vi "Test.vi"() -> ()   [LabVIEW 2013]
uses:
  <resource>/Framework/Providers/lveio/public/EIOAttr.ctl
panel:
  out "Type GUID 2":string
  out "Type GUID":string
  out "Type String 2":string
  out "Array 2":string[](array[string])
  out "properties":T1[](array[typedef])
  out "Array":string[](array[string])
  out "Value":variant
  out "Is Persistent":bool
  out "Tag:Get Names":string[](array[string])
  out "Type String":string
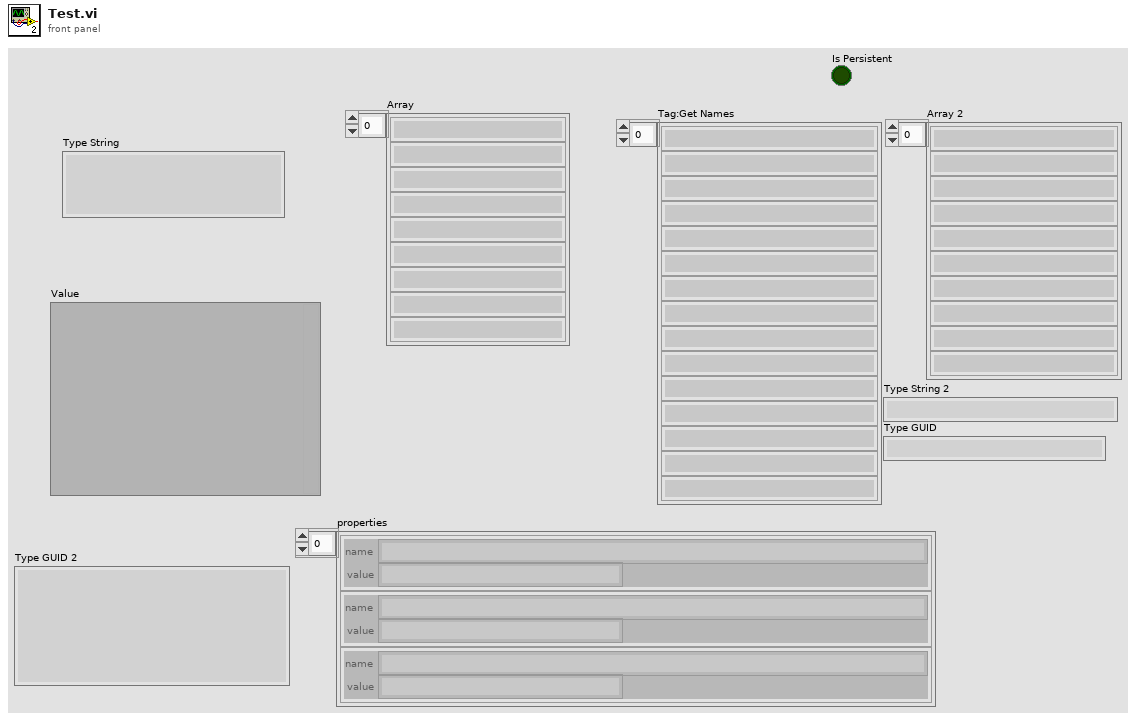
[diagram p1: front panel]
types:
  T1 = typedef "EIOAttr.ctl" = cluster{"name":string, "value":string}
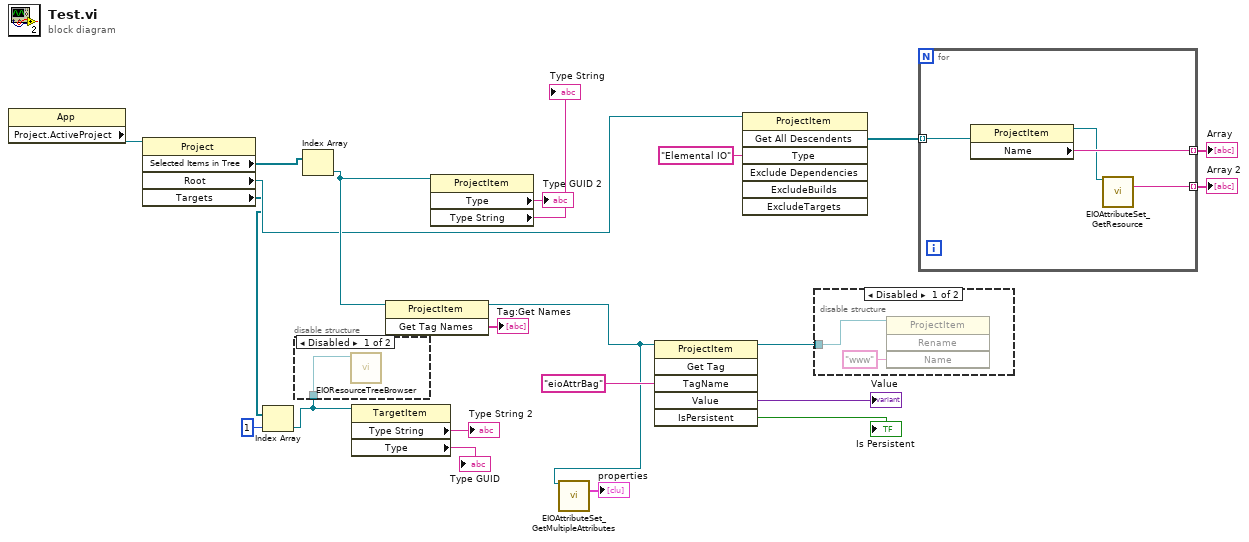
[diagram p0: block diagram]
diagram:
  n1 = property class="App"() -> ("Project.ActiveProject"=w22:refnum<vi>)  [unwired: 2 in, 2 out]
  n2 = property class="Project"(reference=w22) -> ("Selected Items in Tree"=w21:refnum<vi>[], "Root"=w14:refnum<vi>, "Targets"=w9:refnum<vi>[])  [unwired: 1 in, 2 out]
  n3 = Index Array(array=w9, index=1) -> (element=w1:refnum<vi>)
  n4 = disable-structure shown="Disabled" {
    disable-tunnel: w1 -> [w23 _]
    frame Disabled {
      n5 = call <resource>:"EIOResourceTreeBrowser.vi"("target"=w23) -> ()  [unwired: 11 in]
    }
    frame Enabled {
    }
  }
  n6 = Index Array(array=w21) -> (element=w20:refnum<vi>)  [unwired: 1 in]
  n7 = property class="TargetItem"(reference=w1) -> ("Type String"=→"Type String 2":string, "Type"=→"Type GUID":string)  [unwired: 1 in, 2 out]
  n8 = invoke class="ProjectItem" method="Get Tag Names"(reference=w20) -> (reference out=w7:refnum<vi>, "Get Tag Names"=→"Tag:Get Names":string[])  [unwired: 2 in, 1 out]
  n9 = property class="ProjectItem"(reference=w20) -> ("Type"=→"Type GUID 2":string, "Type String"=→"Type String":string)  [unwired: 1 in, 2 out]
  n10 = call <resource>:"EIOAttributeSet_GetMultipleAttributes.vi"("EIOItem Refnum In"=w7) -> ("properties"=→"properties":T1[])  [unwired: 12 in, 2 out]
  n11 = invoke class="ProjectItem" method="Get Tag"(reference=w7, "TagName"="eioAttrBag" ("Tag Name")) -> (reference out=w6:refnum<vi>, "Value"=→"Value":variant, "IsPersistent"=→"Is Persistent":bool)  [unwired: 4 in, 3 out]
  n12 = invoke class="ProjectItem" method="Get All Descendents"(reference=w14, "Type"="Elemental IO") -> ("All Descendents"=w12:refnum<vi>[])  [unwired: 5 in, 6 out]
  n13 = disable-structure shown="Disabled" {
    disable-tunnel: w6 -> [w25 _]
    frame Disabled {
      n14 = invoke class="ProjectItem" method="Rename"(reference=w25, "Name"="www") -> ()  [unwired: 2 in, 4 out]
    }
    frame Enabled {
    }
  }
  n15 = for {
    tunnel: w12 -> [w29] mode=indexing
    tunnel: [w28] -> w11 mode=indexing
    tunnel: [w26] -> w5 mode=indexing
    n16 = property class="ProjectItem"(reference=w29) -> (reference out=w27:refnum<vi>, "Name"=w28:string)  [unwired: 1 in, 1 out]
    n17 = call <resource>:"EIOAttributeSet_GetResource.vi"("EIOItem Refnum In"=w27) -> ("resource name"=w26:string)  [unwired: 9 in, 5 out]
  }
  "Array" <- w11
  "Array 2" <- w5
